vi "Mapping v10.5.0.vi"(5 "Simulate Spectra":bool, 7 "Simulate Drive":bool, 11 "Input Parameters":T6={"Drive Connection Settings"={"Objective GPIB-Port"=1, "Stage GPIB-Port"=0, "Drive Selector"=5, "Drive Velocity (V/s)"=1.0}, "ITC503 Current Values"={"ITC503 Heater"=4.0, "ITC503 Temperature"=4.0, "ITC503 P"=0.0, "ITC503 I"=5.0, "ITC503 D"=0.0, "ITC503 Setpoint"=0.0, "ITC503 Gradient"=0.0, "ITC503 Heater Auto"=FALSE, "ITC503 PID Auto"=FALSE}, "Wavelengths (nm)"=[], "Drive Current Values"={"Voltages"={"Drive X Voltage"=0.0, "Drive Y Voltage"=0.0, "Drive Z Voltage"=0.0}, "Position"={"Drive X Position"=0.0, "Drive Y Position"=0.0, "Drive Z Position"=0.0}}, "iHR Current Values"={"iHR 550 Front Entrance"=0.0, "iHR550 Side Exit"=0.0, "iHR550 Wavelength"=897.9988, "iHR550 Exit Mirror"=2, "iHR550 Grating"="1", "Grating Index"=1}, "Spectra Settings"={"Integration Time"=0.0, "Repetitions"=0, "Mapping Spectra"=TRUE}, "CCD3500 Temperature"=0.0, "Simulate Drive"=FALSE, "Simulate Spectra"=FALSE, "JYCCDLib.IJYCCDReqd"=refnum} {"Drive Connection Settings"."Drive Velocity (V/s)" min=10.0 max=160.0 step=0.1 format="%.1f"; "Drive Connection Settings"."Drive Selector" items=["Obj.", "Stage"]; "Drive Connection Settings"."Stage GPIB-Port" min=1 max=20 step=1 format="%#.0f"; "Drive Connection Settings"."Objective GPIB-Port" min=1 max=20 step=1 format="%#.0f"; "ITC503 Current Values"."ITC503 Gradient" format="%.2f"; "ITC503 Current Values"."ITC503 Setpoint" min=-273.0 max=300000.0 step=0.0001 format="%.1f"; "ITC503 Current Values"."ITC503 I" format="%_1f"; "ITC503 Current Values"."ITC503 P" format="%_1f"; "ITC503 Current Values"."ITC503 Temperature" min=0.0 max=1645.0 step=1e-05 format="%.2f"; "ITC503 Current Values"."ITC503 Heater" min=0.0 max=100.0 step=0.01 scale=0.0..100.0; "Drive Current Values"."Position"."Drive Z Position" min=-273.0 max=300000.0 step=0.0001 format="%.1f"; "Drive Current Values"."Position"."Drive Y Position" min=-273.0 max=300000.0 step=0.0001 format="%.1f"; "Drive Current Values"."Position"."Drive X Position" min=-273.0 max=300000.0 step=0.0001 format="%.1f"; "Drive Current Values"."Voltages"."Drive Z Voltage" min=-273.0 max=300000.0 step=0.0001 format="%.1f"; "Drive Current Values"."Voltages"."Drive Y Voltage" min=-273.0 max=300000.0 step=0.0001 format="%.1f"; "Drive Current Values"."Voltages"."Drive X Voltage" min=-273.0 max=300000.0 step=0.0001 format="%.1f"; "iHR Current Values"."iHR550 Exit Mirror" items=["EntranceMirror", "ExitMirror", "Front", "Side"]; "Spectra Settings"."Repetitions" min=1 max=100 step=1; "Spectra Settings"."Integration Time" min=0.5 max=6000.0 step=1.0 format="%.1f"}) -> ()   [LabVIEW 2010]
uses:
  ESA-C/TypeDefs/ESA-C Connection Settings.ctl
  TypeDefs/Mapping Spectra Params.ctl
  TypeDefs/Mapping Drive Params.ctl
  ESA-C/TypeDefs/ESA-C Set Positions.ctl
  ESA-C/TypeDefs/ESA-C Current Values.ctl
  iHR550/TypeDefs/iHR Current Values.ctl
  ITC503/TypeDefs/ITC503 Current Values.ctl
  TypeDefs/Mapping Input Parameters.ctl
  <vilib>/Utility/miscctls.llb/LVPointTypeDef.ctl
  Global Variables.vi
panel:
  out "JYCCDLib.IJYCCDReqd":refnum<k7>
  out "AutoClose":bool
  out "ITC503 Temperature":dbl caption="Sample (K)" min=10.0 max=160.0 step=0.1 format="%.1f"
  out "CCD3500 Temperature":dbl caption="CCD (°C)" min=10.0 max=160.0 step=0.1 format="%.1f"
  in  "CCD3000 Current Rep.":string="0/0"
  in  "Pause":bool
  out "Current Position":T1 {"Position"."Drive Z Position" min=-273.0 max=300000.0 step=0.0001 format="%.1f"; "Position"."Drive Y Position" min=-273.0 max=300000.0 step=0.0001 format="%.1f"; "Position"."Drive X Position" min=-273.0 max=300000.0 step=0.0001 format="%.1f"; "Voltages"."Drive Z Voltage" min=-273.0 max=300000.0 step=0.0001 format="%.1f"; "Voltages"."Drive Y Voltage" min=-273.0 max=300000.0 step=0.0001 format="%.1f"; "Voltages"."Drive X Voltage" min=-273.0 max=300000.0 step=0.0001 format="%.1f"}
  out "Target Position":T2={"Drive X Set"=10.0, "Drive Y Set"=10.0, "Drive Z Set"=10.0} {"Drive X Set" min=10.0 max=160.0 step=0.1 format="%.1f"; "Drive Z Set" min=10.0 max=160.0 step=0.1 format="%.1f"; "Drive Y Set" min=10.0 max=160.0 step=0.1 format="%.1f"}
  out "Progress":u8(slide) max=10 scale=0.0..100.0
  out "Objective Running":bool caption="Obj."
  out "CCD Running":bool caption="CCD"
  in  "Save Map":bool
  in  "Spectra Params":T3={"Integration Time"=10.0, "Repetitions"=10, "Mapping Spectra"=TRUE} {"Repetitions" min=1 max=100 step=1; "Integration Time" min=0.5 max=6000.0 step=1.0 format="%.1f"}
  in  "Drive Settings":T4={"Objective GPIB-Port"=4, "Stage GPIB-Port"=4, "Drive Selector"=0, "Drive Velocity (V/s)"=5.0} {"Drive Velocity (V/s)" min=10.0 max=160.0 step=0.1 format="%.1f"; "Drive Selector" items=["Obj.", "Stage"]; "Stage GPIB-Port" min=1 max=20 step=1 format="%#.0f"; "Objective GPIB-Port" min=1 max=20 step=1 format="%#.0f"}
  in  "Z Position":dbl caption="Z (µm)" min=0.0 max=100.0 step=0.1 format="%.1f"
  in  "Mapping Params":T5={"X Start Position"=0.0, "X Stop Position"=10.0, "Y Start Position"=0.0, "Y Stop Position"=10.0, "Step Size"=1.0} {"Step Size" min=0.1 max=30.0 step=0.1 format="%.1f"; "Y Stop Position" min=0.0 max=30.0 step=0.1 format="%.1f"; "Y Start Position" min=0.0 max=30.0 step=0.1 format="%.1f"; "X Stop Position" min=0.0 max=30.0 step=0.1 format="%.1f"; "X Start Position" min=0.0 max=30.0 step=0.1 format="%.1f"}
  in  "Exit":bool
  out "Measuring":bool
  in  "Start":bool
  out "Filename":string
  out "Full Data":dbl[][](array[numeric])
  out "Live Data":dbl[][](array[numeric])
  in  "ITC503 Current Values":T7 {"ITC503 Gradient" format="%.2f"; "ITC503 Setpoint" min=-273.0 max=300000.0 step=0.0001 format="%.1f"; "ITC503 I" format="%_1f"; "ITC503 P" format="%_1f"; "ITC503 Temperature" min=0.0 max=1645.0 step=1e-05 format="%.2f"; "ITC503 Heater" min=0.0 max=100.0 step=0.01 scale=0.0..100.0}
  in  "iHR Current Values":T8={"iHR 550 Front Entrance"=0.0, "iHR550 Side Exit"=0.0, "iHR550 Wavelength"=897.9988, "iHR550 Exit Mirror"=2, "iHR550 Grating"="1", "Grating Index"=1} {"iHR550 Exit Mirror" items=["EntranceMirror", "ExitMirror", "Front", "Side"]}
  in  "Wavelengths (nm)":dbl[](array[numeric])
  # "Status"
  # "Active"
  # "Target"
  # "Current"
  # "Parameters"
  # "Spectral"
  # "Spectral / Video Mapping"
  # "Mapping"
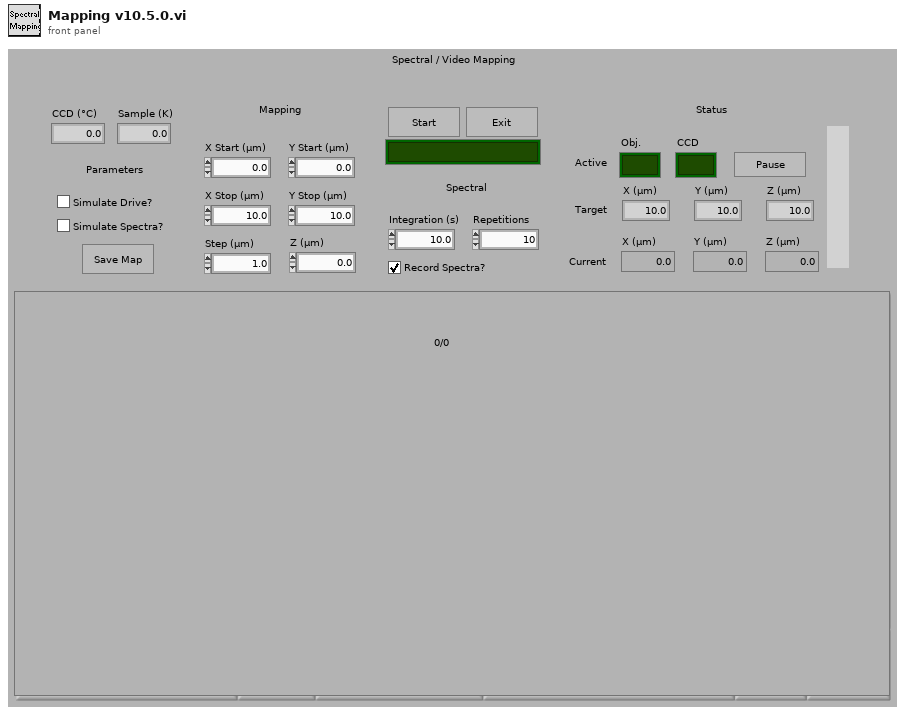
[diagram p1: front panel]
types:
  T1 = typedef "ESA-C Current Values.ctl" = cluster{"Voltages":cluster{"Drive X Voltage":dbl, "Drive Y Voltage":dbl, "Drive Z Voltage":dbl}, "Position":cluster{"Drive X Position":dbl, "Drive Y Position":dbl, "Drive Z Position":dbl}}
  T2 = typedef "ESA-C Set Positions.ctl" = cluster{"Drive X Set":dbl, "Drive Y Set":dbl, "Drive Z Set":dbl}
  T3 = typedef "Mapping Spectra Params.ctl" = cluster{"Integration Time":dbl, "Repetitions":u16, "Mapping Spectra":bool}
  T4 = typedef "ESA-C Connection Settings.ctl" = cluster{"Objective GPIB-Port":i32, "Stage GPIB-Port":i32, "Drive Selector":u16, "Drive Velocity (V/s)":dbl}
  T5 = typedef "Mapping Drive Params.ctl" = cluster{"X Start Position":dbl, "X Stop Position":dbl, "Y Start Position":dbl, "Y Stop Position":dbl, "Step Size":dbl}
  T6 = typedef "Mapping Input Parameters.ctl" = cluster{"Drive Connection Settings":T4, "ITC503 Current Values":T7, "Wavelengths (nm)":dbl[], "Drive Current Values":T1, "iHR Current Values":T8, "Spectra Settings":T3, "CCD3500 Temperature":dbl, "Simulate Drive":bool, "Simulate Spectra":bool, "JYCCDLib.IJYCCDReqd":refnum<k7>}
  T7 = typedef "ITC503 Current Values.ctl" = cluster{"ITC503 Heater":dbl, "ITC503 Temperature":dbl, "ITC503 P":dbl, "ITC503 I":dbl, "ITC503 D":dbl, "ITC503 Setpoint":dbl, "ITC503 Gradient":dbl, "ITC503 Heater Auto":bool, "ITC503 PID Auto":bool}
  T8 = typedef "iHR Current Values.ctl" = cluster{"iHR 550 Front Entrance":dbl, "iHR550 Side Exit":dbl, "iHR550 Wavelength":dbl, "iHR550 Exit Mirror":i32, "iHR550 Grating":string, "Grating Index":i32}
  T9 = typedef "LVPointTypeDef.ctl" = cluster{"Horizontal":i16, "Vertical":i16}
  T10 = typedef "NPC3SG Set Positions.ctl" = cluster{"Drive X Set":dbl, "Drive Y Set":dbl, "Drive Z Set":dbl}
  T11 = cluster{"Intensities":dbl[], "Wavelengths":dbl[]}[]
  T12 = cluster{"Intensities":dbl[], "Wavelengths":dbl[]}
  T13 = enum32{"invalid app kind", "Development System", "Run Time System", "Student Edition", "Embedded LabVIEW", "Evaluation", "Custom"}
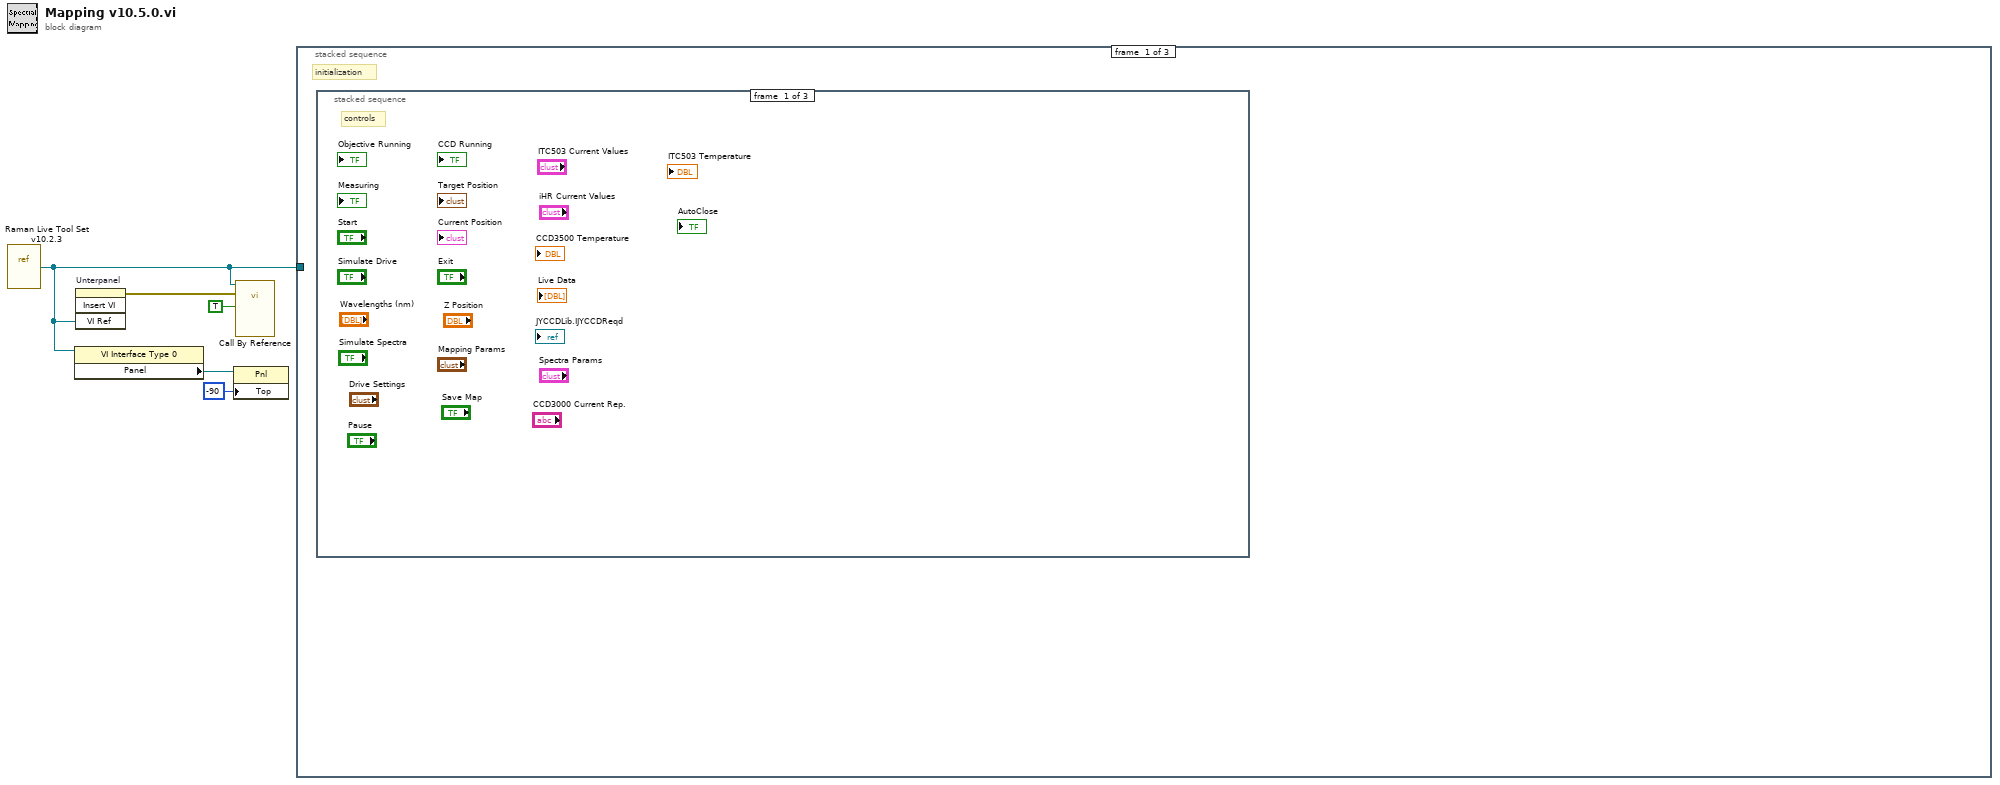
[diagram p0: block diagram]
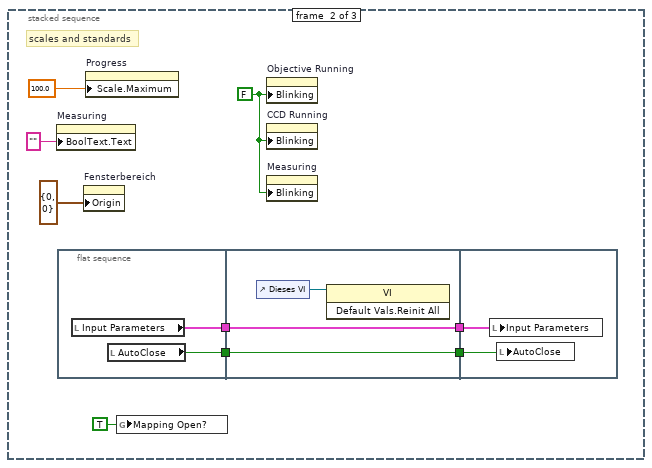
[diagram p2: hidden frame]
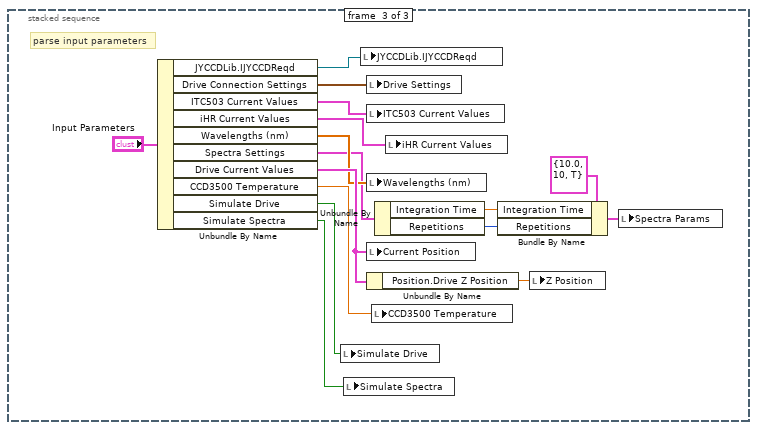
[diagram p3: hidden frame]
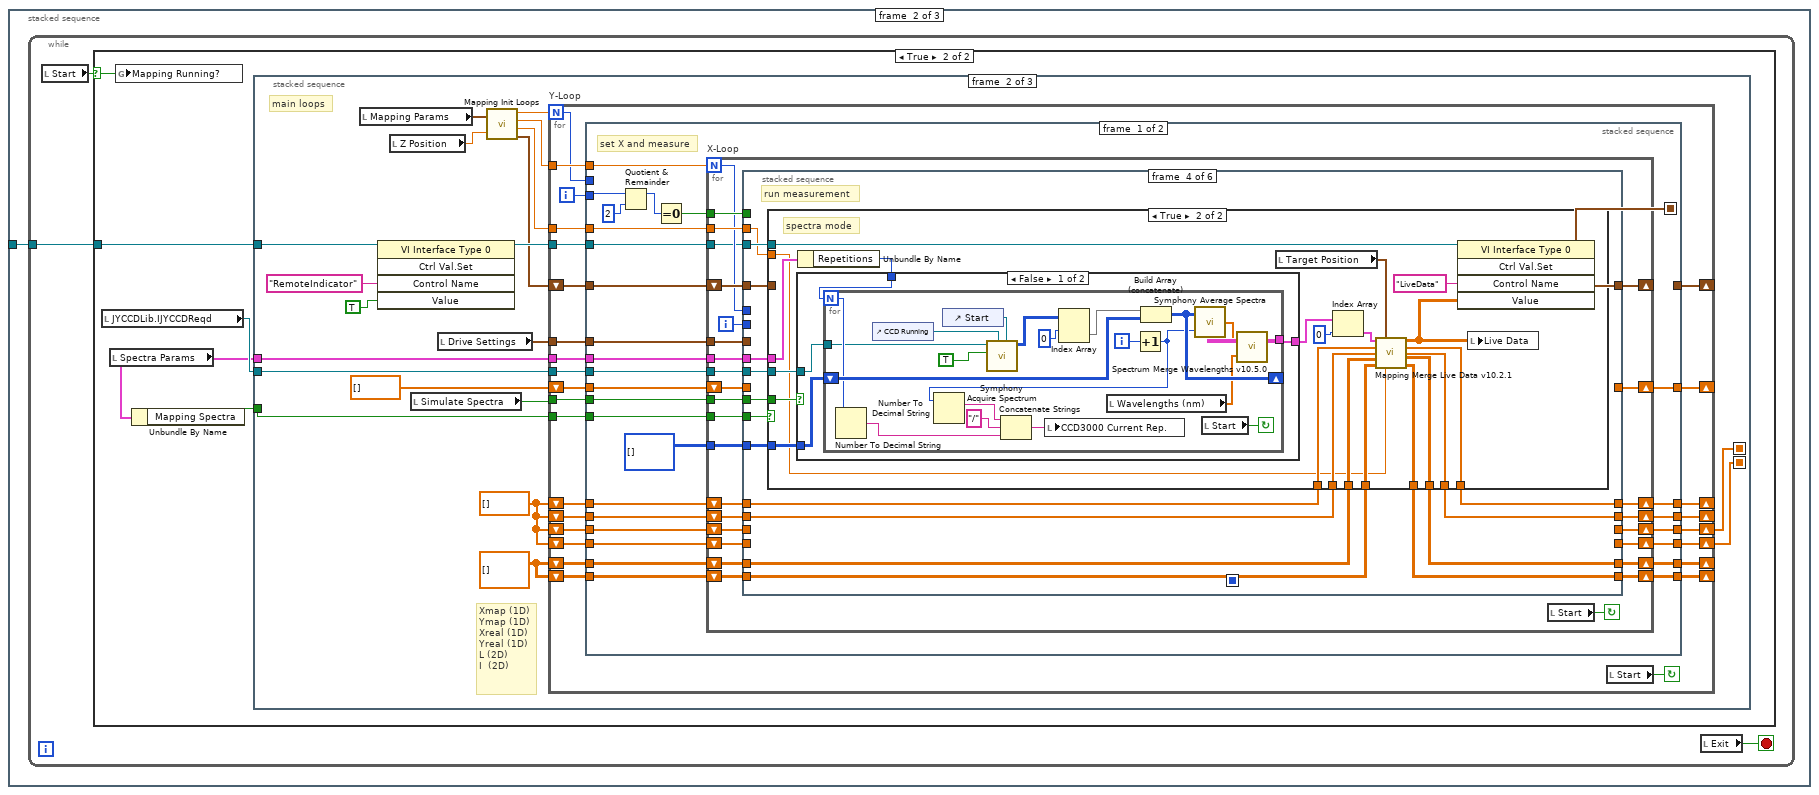
[diagram p4: hidden frame]
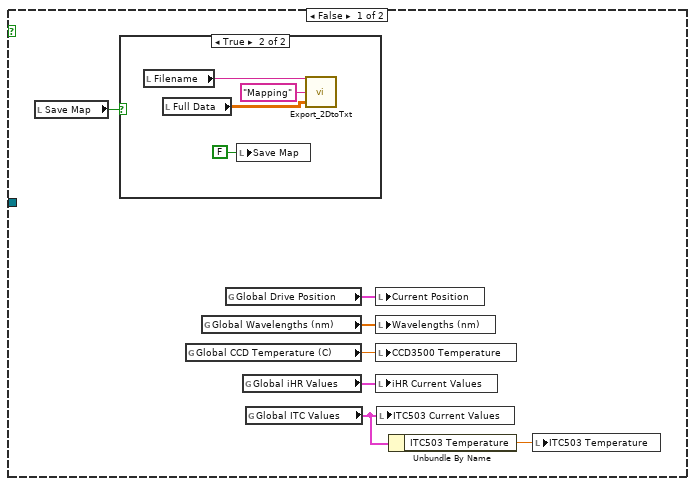
[diagram p5: hidden frame]
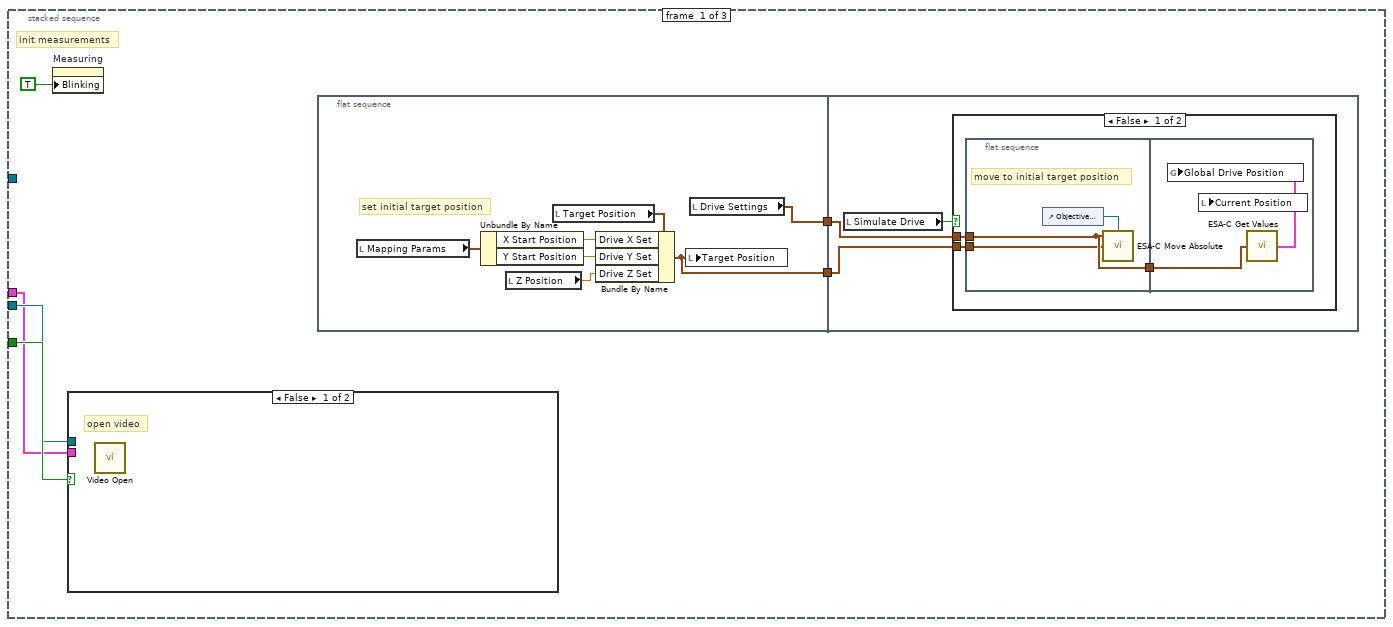
[diagram p7: hidden frame]
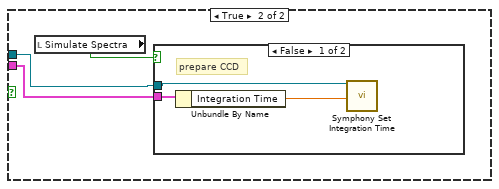
[diagram p9: hidden frame]
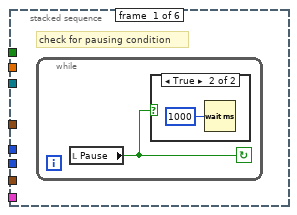
[diagram p11: hidden frame]
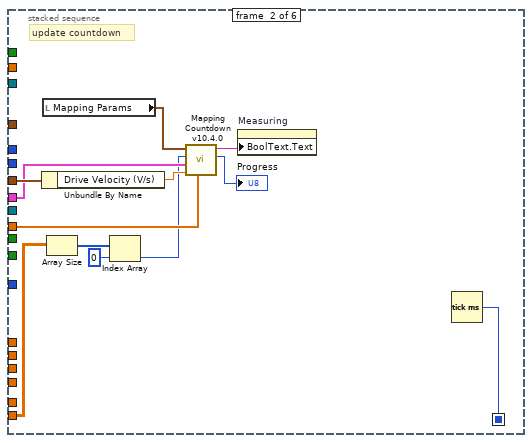
[diagram p13: hidden frame]
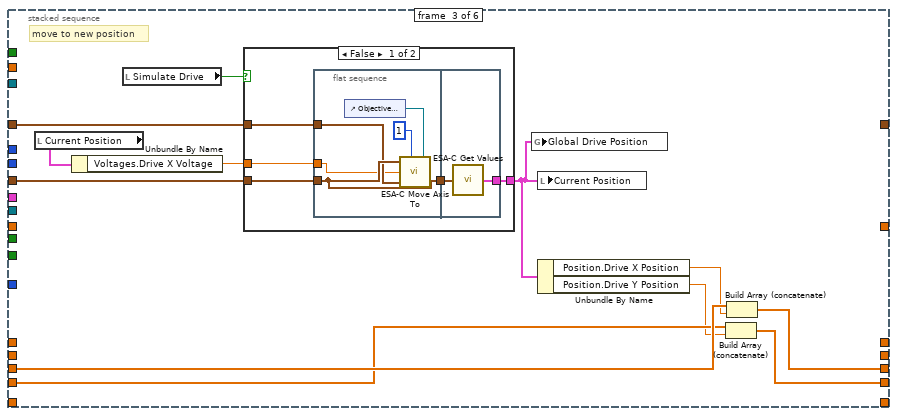
[diagram p14: hidden frame]
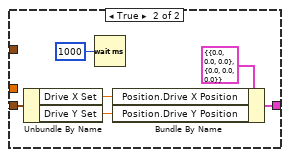
[diagram p15: hidden frame]
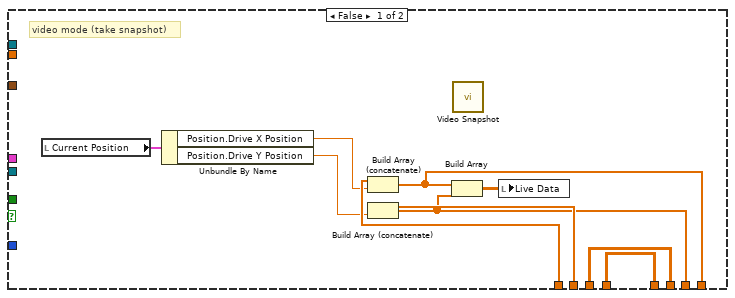
[diagram p16: hidden frame]
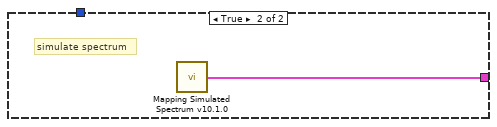
[diagram p17: hidden frame]
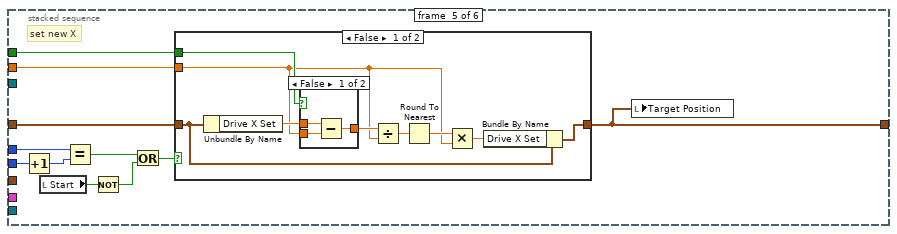
[diagram p18: hidden frame]
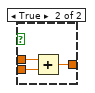
[diagram p19: hidden frame]
diagram:
  n1 = vi-ref "Raman Live Tool Set v10.2.3.vi"() -> (w3:refnum<vi>)
  n2 = property class="VI Interface Type 0"(reference=w3) -> ("Panel"=w2:refnum<vi>)  [unwired: 1 in, 2 out]
  n3 = invoke on="Unterpanel" class="Unterpanel" method="Insert VI"("VI Ref"=w3) -> (error out=w5:errorcluster)  [unwired: 3 in, 3 out]
  n4 = property class="Pnl"(reference=w2, "Top"=-90 ("Position:Oben")) -> ()  [unwired: 1 in, 2 out]
  n5 = call-by-ref "?"(reference=w3, error in=w5, "RemoteIndicator"=TRUE) -> ()  [unwired: 3 in, 2 out]
  n6 = stacked-sequence {
    tunnel: w3 -> [_ w38 w398]
    frame #0 {
      # "initialization"
      n7 = stacked-sequence {
        frame #0 {
          # "controls"
        }
        frame #1 {
          w12 = FALSE ("Blinkend")
          # "scales and standards"
          n8 = property on="Measuring" class="Bool (strict)"("BoolText.Text"="" ("Boolescher Text.Text")) -> ()  [unwired: 2 in, 2 out]
          n9 = flat-sequence {
            tunnel: [w16] -> w9
            tunnel: [w15] -> w6
            tunnel: [w18] -> w10
            tunnel: w9 -> [w18]
            tunnel: [w17] -> w7
            tunnel: w6 -> [w17]
            tunnel: w10 -> [w21]
            tunnel: w7 -> [w20]
            frame #0 {
              n10 = local read "Input Parameters"() -> (w16:T6)
              n11 = local read "AutoClose"() -> (w15:bool)
            }
            frame #1 {
              n12 = control-ref of="Dieses VI"() -> (w19:refnum<vi>)
              n13 = invoke class="VI" method="Default Vals.Reinit All"(reference=w19) -> ()  [unwired: 2 in, 3 out]
            }
            frame #2 {
              n14 = local write "Input Parameters"(w21) -> ()
              n15 = local write "AutoClose"(w20) -> ()
            }
          }
          n16 = property on="Fensterbereich" class="Pane"("Origin"=T9 {"Horizontal"=0, "Vertical"=0}) -> ()  [unwired: 2 in, 2 out]
          n17 = property on="Progress" class="Slide (strict)"("Scale.Maximum"=100.0 ("Skalierung.Bereich:Maximum")) -> ()  [unwired: 2 in, 2 out]
          n18 = global write "Global Variables.vi" "Mapping Open?"(TRUE ("Mapping Open?")) -> ()
          n19 = property on="Objective Running" class="Bool (strict)"("Blinking"=w12) -> ()  [unwired: 2 in, 2 out]
          n20 = property on="CCD Running" class="Bool (strict)"("Blinking"=w12) -> ()  [unwired: 2 in, 2 out]
          n21 = property on="Measuring" class="Bool (strict)"("Blinking"=w12) -> ()  [unwired: 2 in, 2 out]
        }
        frame #2 {
          # "parse input parameters"
          n22 = Unbundle By Name("Input Parameters") -> ("JYCCDLib.IJYCCDReqd"=w22:refnum<k7>, "Drive Connection Settings"=w35:T4, "ITC503 Current Values"=w36:T7, "iHR Current Values"=w26:T8, "Wavelengths (nm)"=w34:dbl[], "Spectra Settings"=w32:T3, "Drive Current Values"=w37:T1, "CCD3500 Temperature"=w27:dbl, "Simulate Drive"=w24:bool, "Simulate Spectra"=w23:bool)
          n23 = local write "Simulate Drive"(w24) -> ()
          n24 = local write "Simulate Spectra"(w23) -> ()
          n25 = local write "JYCCDLib.IJYCCDReqd"(w22) -> ()
          n26 = local write "Drive Settings"(w35) -> ()
          n27 = local write "ITC503 Current Values"(w36) -> ()
          n28 = local write "Wavelengths (nm)"(w34) -> ()
          n29 = local write "Current Position"(w37) -> ()
          n30 = Unbundle By Name(w37) -> ("Position.Drive Z Position"=w33:dbl)
          n31 = local write "CCD3500 Temperature"(w27) -> ()
          n32 = Unbundle By Name(w32) -> ("Integration Time"=w30:dbl, "Repetitions"=w29:u16)
          n33 = local write "iHR Current Values"(w26) -> ()
          n34 = Bundle By Name(cluster=T3 {"Integration Time"=10.0, "Repetitions"=10, "Mapping Spectra"=TRUE} ("Mapping Spectra Settings"), "Integration Time"=w30, "Repetitions"=w29) -> (w28:T3)
          n35 = local write "Z Position"(w33) -> ()
          n36 = local write "Spectra Params"(w28) -> ()
        }
      }
    }
    frame #1 {
      n37 = while {
        tunnel: w38 -> [w41]
        stop <- w40 stop-if-true
        n38 = local read "Start"() -> (w39:bool)
        n39 = case shown="True" w39 {
          selector: w39 -> [_ w53]
          tunnel: w41 -> [_ w57]
          frame False {
            n40 = local read "Save Map"() -> (w48:bool)
            n41 = case shown="True" w48 {
              frame False {
              }
              frame True {
                n42 = local read "Filename"() -> (w51:string)
                n43 = local read "Full Data"() -> (w49:dbl[][])
                n44 = local write "Save Map"(FALSE ("Save Map")) -> ()
                n45 = call "Export_2DtoTxt.vi"("Data (2D)"=w49, "Export Type"="Mapping", "Filename"=w51) -> ()  [unwired: 3 in]
              }
            }
            n46 = global read "Global Variables.vi" "Global CCD Temperature (C)"() -> (w47:dbl)
            n47 = global read "Global Variables.vi" "Global Wavelengths (nm)"() -> (w45:dbl[])
            n48 = global read "Global Variables.vi" "Global Drive Position"() -> (w46:T1)
            n49 = global read "Global Variables.vi" "Global iHR Values"() -> (w44:T8)
            n50 = global read "Global Variables.vi" "Global ITC Values"() -> (w43:T7)
            n51 = local write "Current Position"(w46) -> ()
            n52 = local write "Wavelengths (nm)"(w45) -> ()
            n53 = local write "CCD3500 Temperature"(w47) -> ()
            n54 = local write "iHR Current Values"(w44) -> ()
            n55 = local write "ITC503 Current Values"(w43) -> ()
            n56 = Unbundle By Name(w43) -> ("ITC503 Temperature"=w42:dbl)
            n57 = local write "ITC503 Temperature"(w42) -> ()
          }
          frame True {
            n58 = local read "JYCCDLib.IJYCCDReqd"() -> (w55:refnum<k7>)
            n59 = local read "Spectra Params"() -> (w54:T3)
            n60 = global write "Global Variables.vi" "Mapping Running?"(w53) -> ()
            n61 = Unbundle By Name(w54) -> ("Mapping Spectra"=w56:bool)
            n62 = stacked-sequence {
              seq-local: [_ w88 _] -> [_ _ w377]
              seq-local: [_ w89 _] -> [_ _ w376]
              tunnel: w57 -> [_ w99 _]
              tunnel: w56 -> [w62 w98 w378]
              tunnel: w54 -> [w60 w96 _]
              tunnel: w55 -> [w61 w95 _]
              frame #0 {
                # "init measurements"
                n63 = property on="Measuring" class="Bool (strict)"("Blinking"=TRUE ("Blinkend")) -> ()  [unwired: 2 in, 2 out]
                n64 = case shown="False" w62 {
                  tunnel: w61 -> [_ w84]
                  tunnel: w60 -> [_ w83]
                  frame False {
                    # "open video"
                    n65 = call "Video Open.vi"() -> ()  [unwired: 11 in, 1 out]
                  }
                  frame True {
                    n66 = local read "Simulate Spectra"() -> (w82:bool)
                    n67 = case shown="False" w82 {
                      tunnel: w84 -> [w87 _]
                      tunnel: w83 -> [w86 _]
                      frame False {
                        # "prepare CCD"
                        n68 = Unbundle By Name(w86) -> ("Integration Time"=w85:dbl)
                        n69 = call "Symphony Set Integration Time.vi"("JYCCDLib.IJYCCDReqd"=w87, "Integration (s)"=w85) -> ()  [unwired: 13 in, 1 out]
                      }
                      frame True {
                      }
                    }
                  }
                }
                n70 = flat-sequence {
                  tunnel: [w65] -> w59
                  tunnel: [w64] -> w58
                  tunnel: w59 -> [w71]
                  tunnel: w58 -> [w72]
                  frame #0 {
                    # "set initial target position"
                    n71 = local read "Mapping Params"() -> (w70:T5)
                    n72 = Unbundle By Name(w70) -> ("X Start Position"=w68:dbl, "Y Start Position"=w67:dbl)
                    n73 = local read "Z Position"() -> (w66:dbl)
                    n74 = local read "Target Position"() -> (w69:T2)
                    n75 = Bundle By Name(cluster=w69, "Drive X Set"=w68, "Drive Y Set"=w67, "Drive Z Set"=w66) -> (w65:T2)
                    n76 = local write "Target Position"(w65) -> ()
                    n77 = local read "Drive Settings"() -> (w64:T4)
                  }
                  frame #1 {
                    n78 = local read "Simulate Drive"() -> (w73:bool)
                    n79 = case shown="False" w73 {
                      tunnel: w72 -> [w76 _]
                      tunnel: w71 -> [w74 _]
                      frame False {
                        n80 = flat-sequence {
                          tunnel: w76 -> [w78]
                          tunnel: [w78] -> w75
                          tunnel: w74 -> [w77]
                          tunnel: w75 -> [w81]
                          frame #0 {
                            # "move to initial target position"
                            n81 = control-ref of="Objective Running"() -> (w79:refnum<vi>)
                            n82 = call "ESA-C Move Absolute.vi"("Running"=w79, "Drive New Abs. Positions"=w77, "Drive Connection Settings"=w78) -> ()  [unwired: 2 in]
                          }
                          frame #1 {
                            n83 = call "ESA-C Get Values.vi"("Drive Connection Settings"=w81) -> ("Drive Current Values"=w80:T1)
                            n84 = global write "Global Variables.vi" "Global Drive Position"(w80) -> ()
                            n85 = local write "Current Position"(w80) -> ()
                          }
                        }
                      }
                      frame True {
                      }
                    }
                  }
                }
              }
              frame #1 {
                w107 = dbl[][] []
                w90 = dbl[] []
                # "main loops"
                # "Xmap (1D)\nYmap (1D)\nXreal (1D)\nYreal (1D)\nL (2D)\nI  (2D)"
                n86 = local read "Mapping Params"() -> (w93:T5)
                n87 = invoke class="VI Interface Type 0" method="Ctrl Val.Set"(reference=w99, "Control Name"="RemoteIndicator" ("Elementname"), "Value"=TRUE) -> (reference out=w101:refnum<vi>)  [unwired: 2 in, 4 out]
                n88 = local read "Z Position"() -> (w92:dbl)
                n89 = local read "Simulate Spectra"() -> (w91:bool)
                n90 = local read "Drive Settings"() -> (w94:T4)
                n91 = call "Mapping Init Loops.vi"("Z Position"=w92, "Mapping Params"=w93) -> ("Start Positions"=w100:T10, "Step Size"=w102:dbl, "X Steps"=w103:dbl, "Y Steps"=w104:dbl)
                n92 = for "Y-Loop" {
                  N: w104 -> [w120]
                  tunnel: w103 -> [w133]
                  tunnel: w102 -> [w132]
                  shift-right: [w118] -> _
                  shift-left: w100 -> [w119]
                  shift-right: [w124] -> _
                  shift-left: w107 -> [w128]
                  shift-right: [w125] -> _
                  shift-left: w107 -> [w129]
                  shift-right: [w127] -> _
                  shift-left: w90 -> [w131]
                  shift-right: [w126] -> _
                  shift-left: w90 -> [w130]
                  tunnel: w101 -> [w122]
                  tunnel: w91 -> [w121]
                  tunnel: w94 -> [w117]
                  tunnel: w98 -> [w116]
                  tunnel: w96 -> [w115]
                  shift-right: [w113] -> _
                  shift-left: dbl[] [] -> [w114]
                  tunnel: w95 -> [w112]
                  shift-right: [w109] -> w89
                  shift-left: w90 -> [w110]
                  shift-right: [w108] -> w88
                  shift-left: w90 -> [w111]
                  i -> [w123]
                  stop <- w134 continue-if-true
                  n93 = stacked-sequence {
                    seq-local: [w148 _] -> [_ w349]
                    tunnel: w133 -> [w163 _]
                    tunnel: w132 -> [w162 w350]
                    tunnel: w131 -> [w161 _]
                    tunnel: w130 -> [w160 _]
                    tunnel: w129 -> [w159 _]
                    tunnel: w128 -> [w135 _]
                    tunnel: [w158 _] -> w127
                    tunnel: [w157 _] -> w126
                    tunnel: [w156 _] -> w125
                    tunnel: [w155 _] -> w124
                    tunnel: w123 -> [w152 w353]
                    tunnel: w122 -> [w150 _]
                    tunnel: w121 -> [w149 _]
                    tunnel: w120 -> [_ w351]
                    tunnel: w119 -> [w147 _]
                    tunnel: [_ w347] -> w118
                    tunnel: w117 -> [w146 w348]
                    tunnel: w116 -> [w145 _]
                    tunnel: w115 -> [w144 _]
                    tunnel: w114 -> [w143 _]
                    tunnel: [w142 _] -> w113
                    tunnel: w112 -> [w141 _]
                    tunnel: w111 -> [w139 _]
                    tunnel: w110 -> [w138 _]
                    tunnel: [w137 _] -> w109
                    tunnel: [w136 _] -> w108
                    frame #0 {
                      # "set X and measure"
                      n94 = Quotient & Remainder(x=w152, y=2) -> (x-y*floor(x/y)=w153:i32)  [unwired: 1 out]
                      n95 = Equal To 0?(x=w153) -> (x = 0?=w151:bool)
                      n96 = for "X-Loop" {
                        N: w163 -> [w177]
                        tunnel: w162 -> [w189]
                        shift-right: [w188] -> w148
                        shift-left: w147 -> [w190]
                        shift-right: [w183] -> w158
                        shift-left: w161 -> [w187]
                        shift-right: [w182] -> w157
                        shift-left: w160 -> [w186]
                        shift-right: [w180] -> w156
                        shift-left: w159 -> [w185]
                        shift-right: [w181] -> w155
                        shift-left: w135 -> [w184]
                        tunnel: w151 -> [w179]
                        tunnel: w150 -> [w176]
                        tunnel: w149 -> [w175]
                        tunnel: w146 -> [w174]
                        tunnel: w145 -> [w173]
                        tunnel: w144 -> [w172]
                        shift-right: [w171] -> w142
                        shift-left: w143 -> [w170]
                        tunnel: w141 -> [w169]
                        tunnel: u16[][] [] -> [w168]
                        shift-right: [w164] -> w136
                        shift-left: w139 -> [w167]
                        shift-right: [w165] -> w137
                        shift-left: w138 -> [w166]
                        i -> [w178]
                        stop <- w191 continue-if-true
                        n97 = stacked-sequence {
                          seq-local: [_ w198 _ _ _ _] -> [_ _ _ _ _ w338]
                          tunnel: w190 -> [_ _ w217 w251 w315 _]
                          tunnel: w189 -> [_ _ _ w236 w313 _]
                          tunnel: [_ _ _ _ w312 _] -> w188
                          tunnel: w187 -> [_ _ _ w250 _ _]
                          tunnel: w186 -> [_ _ _ w249 _ _]
                          tunnel: w185 -> [_ _ _ w247 _ _]
                          tunnel: w184 -> [_ w197 _ w248 _ _]
                          tunnel: [_ _ _ w246 _ _] -> w183
                          tunnel: [_ _ _ w245 _ _] -> w182
                          tunnel: [_ _ _ w244 _ _] -> w181
                          tunnel: [_ _ _ w243 _ _] -> w180
                          tunnel: w179 -> [_ _ _ _ w314 _]
                          tunnel: w178 -> [_ _ _ _ w318 _]
                          tunnel: w177 -> [_ _ _ _ w316 _]
                          tunnel: w176 -> [_ _ _ w242 _ _]
                          tunnel: w175 -> [_ _ _ w241 _ _]
                          tunnel: w174 -> [_ w201 w215 _ _ _]
                          tunnel: w173 -> [_ _ _ w240 _ _]
                          tunnel: w172 -> [_ w200 _ w238 _ _]
                          tunnel: [_ _ _ _ _ w335] -> w171
                          tunnel: w170 -> [_ w199 _ _ _ w337]
                          tunnel: w169 -> [_ _ _ w239 _ _]
                          tunnel: w168 -> [_ _ _ w237 _ _]
                          tunnel: w167 -> [_ _ w212 _ _ _]
                          tunnel: w166 -> [_ _ w211 _ _ _]
                          tunnel: [_ _ w208 _ _ _] -> w165
                          tunnel: [_ _ w207 _ _ _] -> w164
                          frame #0 {
                            # "check for pausing condition"
                            n98 = while {
                              stop <- w192 continue-if-true
                              n99 = local read "Pause"() -> (w192:bool)
                              n100 = case shown="True" w192 {
                                frame False {
                                }
                                frame True {
                                n101 = Wait (ms)(milliseconds to wait=u32 1000) -> ()  [unwired: 1 out]
                                }
                              }
                            }
                          }
                          frame #1 {
                            # "update countdown"
                            n102 = Unbundle By Name(w201) -> ("Drive Velocity (V/s)"=w202:dbl)
                            n103 = local read "Mapping Params"() -> (w205:T5)
                            n104 = Array Size(array=w197) -> (size(s)=w196:i32[])
                            n105 = Index Array(array=w196, index=0) -> (element=w194:i32)
                            n106 = call "Mapping Countdown v10.4.0.vi"("Execution Times (s)"=w199, "Drive Velocity"=w202, "Mapping Spectra Settings"=w200, "Ready Steps"=w194, "Mapping Drive Parameters"=w205) -> ("Progress"=→"Progress":i16, "Time String"=w203:string)  [unwired: 5 in]
                            n107 = property on="Measuring" class="Bool (strict)"("BoolText.Text"=w203) -> ()  [unwired: 2 in, 2 out]
                            n108 = Tick Count (ms)() -> (millisecond timer value=w198:u32)
                          }
                          frame #2 {
                            # "move to new position"
                            n109 = local read "Current Position"() -> (w214:T1)
                            n110 = Unbundle By Name(w214) -> ("Voltages.Drive X Voltage"=w213:dbl)
                            n111 = local read "Simulate Drive"() -> (w216:bool)
                            n112 = case shown="False" w216 {
                              tunnel: w217 -> [w221 w234]
                              tunnel: [w220 w231] -> w206
                              tunnel: w215 -> [w219 _]
                              tunnel: w213 -> [w218 _]
                              frame False {
                                n113 = flat-sequence {
                                tunnel: w221 -> [w226]
                                tunnel: [w227] -> w222
                                tunnel: w219 -> [w227]
                                tunnel: w218 -> [w223]
                                tunnel: w222 -> [w229]
                                tunnel: [w228] -> w220
                                frame #0 {
                                n114 = control-ref of="Objective Running"() -> (w224:refnum<vi>)
                                n115 = call "ESA-C Move Axis To.vi"("Drive Connection Settings"=w227, "Axis"=1, "Current Voltage (V)"=w223, "Drive New Abs. Positions"=w226, "Running"=w224) -> ()  [unwired: 2 in]
                                }
                                frame #1 {
                                n116 = call "ESA-C Get Values.vi"("Drive Connection Settings"=w229) -> ("Drive Current Values"=w228:T1)
                                }
                                }
                              }
                              frame True {
                                n117 = Unbundle By Name(w234) -> ("Drive X Set"=w235:dbl, "Drive Y Set"=w232:dbl)
                                n118 = Wait (ms)(milliseconds to wait=u32 1000 ("Zu wartende ms")) -> ()  [unwired: 1 out]
                                n119 = Bundle By Name(cluster=T1 {"Voltages"={"Drive X Voltage"=0.0, "Drive Y Voltage"=0.0, "Drive Z Voltage"=0.0}, "Position"={"Drive X Position"=0.0, "Drive Y Position"=0.0, "Drive Z Position"=0.0}} ("Drive Current Values"), "Position.Drive X Position"=w235, "Position.Drive Y Position"=w232) -> (w231:T1)
                              }
                            }
                            n120 = global write "Global Variables.vi" "Global Drive Position"(w206) -> ()
                            n121 = local write "Current Position"(w206) -> ()
                            n122 = Unbundle By Name(w206) -> ("Position.Drive X Position"=w210:dbl, "Position.Drive Y Position"=w209:dbl)
                            n123 = Build Array (concatenate)(w211, w209) -> (w208:dbl[])
                            n124 = Build Array (concatenate)(w212, w210) -> (w207:dbl[])
                          }
                          frame #3 {
                            # "run measurement"
                            n125 = case shown="True" w240 {
                              tunnel: w251 -> [_ _]
                              tunnel: w250 -> [w258 w279]
                              tunnel: w249 -> [w257 w278]
                              tunnel: w248 -> [w260 w276]
                              tunnel: w247 -> [w261 w277]
                              tunnel: [w255 w273] -> w246
                              tunnel: [w256 w272] -> w245
                              tunnel: [w260 w275] -> w244
                              tunnel: [w261 w274] -> w243
                              tunnel: w242 -> [_ w281]
                              tunnel: w241 -> [_ w280]
                              tunnel: w239 -> [_ w269]
                              tunnel: w238 -> [_ w268]
                              tunnel: w237 -> [_ w266]
                              tunnel: w236 -> [_ w262]
                              frame False {
                                # "video mode (take snapshot)"
                                n126 = local read "Current Position"() -> (w259:T1)
                                n127 = Unbundle By Name(w259) -> ("Position.Drive X Position"=w254:dbl, "Position.Drive Y Position"=w253:dbl)
                                n128 = Build Array (concatenate)(w258, w254) -> (w255:dbl[])
                                n129 = Build Array (concatenate)(w257, w253) -> (w256:dbl[])
                                n130 = Build Array(w255, w256) -> (w252:dbl[][])
                                n131 = call "Video Snapshot.vi"() -> ()  [unwired: 11 in, 1 out]
                                n132 = local write "Live Data"(w252) -> ()
                              }
                              frame True {
                                # "spectra mode"
                                n133 = Unbundle By Name(w268) -> ("Repetitions"=w267:u16)
                                n134 = case shown="False" w280 {
                                tunnel: [w285 w307] -> w265
                                tunnel: w269 -> [w286 _]
                                tunnel: w267 -> [w284 _]
                                tunnel: w266 -> [w283 _]
                                frame False {
                                n135 = for {
                                N: w284 -> [w293]
                                shift-right: [w304] -> _
                                shift-left: w283 -> [w305]
                                tunnel: [w302] -> w285
                                tunnel: w286 -> [w291]
                                i -> [w306]
                                stop <- w300 continue-if-true
                                n136 = Number To Decimal String(number=w293) -> (decimal integer string=w296:string)  [unwired: 1 in]
                                n137 = control-ref of="CCD Running"() -> (w299:refnum<vi>)
                                n138 = control-ref of="Start"() -> (w298:refnum<vi>)
                                n139 = call "Symphony Acquire Spectrum.vi"("Acquire"=w298, "Running"=w299, "ShutterOpen"=TRUE, "JYCCDLib.IJYCCDReqd"=w291) -> ("Raw Data"=w288:i32[][])  [unwired: 6 in, 1 out]
                                n140 = Index Array(array=w288, index (row)=0) -> (element=w287:i32[])  [unwired: 1 in]
                                n141 = local read "Wavelengths (nm)"() -> (w301:dbl[])
                                n142 = Increment(x=w306) -> (x+1=w292:i32)
                                n143 = Number To Decimal String(number=w292) -> (decimal integer string=w295:string)  [unwired: 1 in]
                                n144 = Concatenate Strings(w295, "/" ("string"), w296) -> (w294:string)
                                n145 = local write "CCD3000 Current Rep."(w294) -> ()
                                n146 = Build Array (concatenate)(w287, w305) -> (w304:i32[][])
                                n147 = call "Symphony Average Spectra.vi"("Repetitions"=w292, "Raw Spectra"=w304) -> ("Raw Spectrum"=w303:dbl[])
                                n148 = local read "Start"() -> (w300:bool)
                                n149 = call "Spectrum Merge Wavelengths v10.5.0.vi"("Wavelengths (nm)"=w301, "Raw Spectrum"=w303) -> ("Spectrum-Cluster"=w302:T11)  [unwired: 1 out]
                                }
                                }
                                frame True {
                                # "simulate spectrum"
                                n150 = call "Mapping Simulated Spectrum v10.1.0.vi"() -> ("Simulated Spectrum"=w307:cluster{i32[], dbl[]}[])
                                }
                                }
                                n151 = local read "Target Position"() -> (w271:T2)
                                n152 = Index Array(array=w265, index=0 ("Index")) -> (element=w264:T12)
                                n153 = call "Mapping Merge Live Data v10.2.1.vi"("New Spectrum"=w264, "Target Position"=w271, "X in (1D)"=w279, "Y in (1D)"=w278, "L in (2D)"=w277, "I in (2D)"=w276, "Step Size"=w262) -> ("Live Data"=w270:dbl[][], "X out (1D)"=w273:dbl[], "Y out (1D)"=w272:dbl[], "L out (2D)"=w274:dbl[][], "I out (2D)"=w275:dbl[][])  [unwired: 4 in]
                                n154 = invoke class="VI Interface Type 0" method="Ctrl Val.Set"(reference=w281, "Control Name"="LiveData" ("Elementname"), "Value"=w270) -> ()  [unwired: 2 in, 5 out]
                                n155 = local write "Live Data"(w270) -> ()
                              }
                            }
                          }
                          frame #4 {
                            # "set new X"
                            n156 = Increment(x=w318) -> (x+1=w317:i32)
                            n157 = local read "Start"() -> (w311:bool)
                            n158 = Equal?(x=w316, y=w317) -> (x = y?=w308:bool)
                            n159 = Not(x=w311) -> (.not. x?=w310:bool)
                            n160 = Or(x=w308, y=w310) -> (x .or. y?=w309:bool)
                            n161 = case shown="False" w309 {
                              tunnel: w315 -> [w326 w334]
                              tunnel: [w325 w334] -> w312
                              tunnel: w314 -> [w324 _]
                              tunnel: w313 -> [w319 _]
                              frame False {
                                n162 = Unbundle By Name(w326) -> ("Drive X Set"=w327:dbl)
                                n163 = case shown="False" w324 {
                                tunnel: w327 -> [w330 w332]
                                tunnel: [w329 w333] -> w320
                                tunnel: w319 -> [w328 w331]
                                frame False {
                                n164 = Subtract(x=w330, y=w328) -> (x-y=w329:dbl)
                                }
                                frame True {
                                n165 = Add(x=w332, y=w331) -> (x+y=w333:dbl)
                                }
                                }
                                n166 = Divide(x=w320, y=w319) -> (x/y=w323:dbl)
                                n167 = Round To Nearest(number=w323) -> (nearest integer value=w322:dbl)
                                n168 = Multiply(x=w322, y=w319) -> (x*y=w321:dbl)
                                n169 = Bundle By Name(cluster=w326, "Drive X Set"=w321) -> (w325:T10)
                              }
                              frame True {
                              }
                            }
                            n170 = local write "Target Position"(w312) -> ()
                          }
                          frame #5 {
                            n171 = Tick Count (ms)() -> (millisecond timer value=w339:u32)
                            n172 = Subtract(x=w339, y=w338) -> (x-y=w341:u32)
                            n173 = Divide(x=w341, y=u32 1000) -> (x/y=w336:dbl)
                            n174 = Build Array (concatenate)(w337, w336) -> (w335:dbl[])
                          }
                        }
                        n175 = local read "Start"() -> (w191:bool)
                      }
                    }
                    frame #1 {
                      # "set new Y\nand move to new position"
                      n176 = Increment(x=w353) -> (x+1=w352:i32)
                      n177 = local read "Start"() -> (w343:bool)
                      n178 = Equal?(x=w351, y=w352) -> (x = y?=w345:bool)
                      n179 = local read "Simulate Drive"() -> (w346:bool)
                      n180 = Not(x=w343) -> (.not. x?=w344:bool)
                      n181 = Or(x=w345, y=w344) -> (x .or. y?=w342:bool)
                      n182 = case shown="False" w342 {
                        tunnel: w349 -> [w374 w375]
                        tunnel: [w373 w375] -> w347
                        tunnel: w350 -> [w368 _]
                        frame False {
                          n183 = Unbundle By Name(w374) -> ("Drive Y Set"=w372:dbl)
                          n184 = Add(x=w368, y=w372) -> (x+y=w369:dbl)
                          n185 = Divide(x=w369, y=w368) -> (x/y=w370:dbl)
                          n186 = Round To Nearest(number=w370) -> (nearest integer value=w371:dbl)
                          n187 = Multiply(x=w371, y=w368) -> (x*y=w367:dbl)
                          n188 = Bundle By Name(cluster=w374, "Drive Y Set"=w367) -> (w373:T10)
                        }
                        frame True {
                        }
                      }
                      n189 = case shown="False" w346 {
                        tunnel: w348 -> [w358 _]
                        tunnel: w347 -> [w357 _]
                        frame False {
                          n190 = local read "Current Position"() -> (w356:T1)
                          n191 = Unbundle By Name(w356) -> ("Voltages.Drive Y Voltage"=w355:dbl)
                          n192 = flat-sequence {
                            tunnel: w358 -> [w360]
                            tunnel: w357 -> [w361]
                            tunnel: w355 -> [w362]
                            tunnel: [w360] -> w359
                            tunnel: [w366] -> w354
                            tunnel: w359 -> [w365]
                            frame #0 {
                              n193 = control-ref of="Objective Running"() -> (w364:refnum<vi>)
                              n194 = call "ESA-C Move Axis To.vi"("Drive Connection Settings"=w360, "Axis"=2, "Current Voltage (V)"=w362, "Drive New Abs. Positions"=w361, "Running"=w364) -> ()  [unwired: 2 in]
                            }
                            frame #1 {
                              n195 = call "ESA-C Get Values.vi"("Drive Connection Settings"=w365) -> ("Drive Current Values"=w366:T1)
                            }
                          }
                          n196 = global write "Global Variables.vi" "Global Drive Position"(w354) -> ()
                          n197 = local write "Current Position"(w354) -> ()
                        }
                        frame True {
                        }
                      }
                      n198 = local write "Target Position"(w347) -> ()
                    }
                  }
                  n199 = local read "Start"() -> (w134:bool)
                }
              }
              frame #2 {
                # "conclude measurement"
                n200 = flat-sequence {
                  tunnel: w377 -> [w385]
                  tunnel: w376 -> [w384]
                  tunnel: w378 -> [w393]
                  frame #0 {
                    # "save data"
                    n201 = global read "Global Variables.vi" "Global CCD Temperature (C)"() -> (w381:dbl)
                    n202 = global read "Global Variables.vi" "Global iHR Values"() -> (w379:T8)
                    n203 = local read "Mapping Params"() -> (w383:T5)
                    n204 = global read "Global Variables.vi" "Global ITC Values"() -> (w380:T7)
                    n205 = local read "Spectra Params"() -> (w388:T3)
                    n206 = Unbundle By Name(w383) -> ("Step Size"=w382:dbl)
                    n207 = local read "Live Data"() -> (w387:dbl[][])
                    n208 = call "Mapping Merge Real Positions v10.2.1.vi"("Live Data In"=w387, "X in (1D)"=w385, "Y in (1D)"=w384, "Step Size"=w382) -> ("Live Data Out"=w386:dbl[][])  [unwired: 11 in]
                    "Full Data" <- w386
                    n209 = call "Export_mappingFileName.vi"("ITC503 Current Values"=w380, "iHR Current Values"=w379, "Spectra Settings"=w388, "Mapping Parameters"=w383, "CCD3500 Temperature"=w381) -> ("Filename"=w389:string)
                    "Filename" <- w389
                    n210 = call "Export_2DtoTxt v10.2.0.vi"("Data (2D)"=w386, "Export Type"="Mapping", "Filename"=w389) -> ()  [unwired: 3 in]
                  }
                  frame #1 {
                    # "reset indicators"
                    n211 = case shown="False" w393 {
                      frame False {
                        n212 = call "Video Close.vi"() -> ()  [unwired: 11 in, 1 out]
                      }
                      frame True {
                      }
                    }
                    n213 = local write "Start"(FALSE ("Start")) -> ()
                    n214 = local write "CCD3000 Current Rep."("0/0" ("CCD3000 Current Rep.")) -> ()
                    n215 = global write "Global Variables.vi" "Mapping Running?"(FALSE ("Mapping Running?")) -> ()
                    n216 = property on="Measuring" class="Bool (strict)"("BoolText.Text"="" ("Boolescher Text.Text")) -> ()  [unwired: 2 in, 2 out]
                    n217 = property on="Measuring" class="Bool (strict)"("Blinking"=FALSE ("Measuring")) -> ()  [unwired: 2 in, 2 out]
                  }
                }
              }
            }
          }
        }
        n218 = local read "Exit"() -> (w40:bool)
      }
    }
    frame #2 {
      n219 = invoke class="VI Interface Type 0" method="Ctrl Val.Set"(reference=w398, "Control Name"="Exit" ("Elementname"), "Value"=TRUE) -> ()  [unwired: 2 in, 5 out]
      n220 = local read "AutoClose"() -> (w397:bool)
      n221 = flat-sequence {
        tunnel: w397 -> [w401]
        frame #0 {
          # "reset and close"
          n222 = control-ref of="Dieses VI"() -> (w404:refnum<vi>)
          n223 = global write "Global Variables.vi" "Mapping Open?"(FALSE ("Mapping Open?")) -> ()
          n224 = invoke class="VI" method="Default Vals.Reinit All"(reference=w404) -> (reference out=w402:refnum<vi>)  [unwired: 2 in, 2 out]
          n225 = property on="Measuring" class="Bool (strict)"("BoolText.Text"="" ("Boolescher Text.Text")) -> ()  [unwired: 2 in, 2 out]
          n226 = property class="App"() -> ("App.Kind"=w405:T13)  [unwired: 2 in, 2 out]
          n227 = case shown="\"Development System\"" w405 {
            tunnel: w402 -> [w407 w409]
            tunnel: w401 -> [_ w408]
            frame "invalid app kind", Default {
              n228 = invoke on="Invoke Node" class="VI" method="FP.Close"(reference=w407) -> ()  [unwired: 2 in, 3 out]
            }
            frame "Development System" {
              n229 = case shown="True" w408 {
                tunnel: w409 -> [_ w410]
                frame False {
                }
                frame True {
                  n230 = invoke on="Invoke Node" class="VI" method="FP.Close"(reference=w410) -> ()  [unwired: 2 in, 3 out]
                }
              }
            }
          }
        }
      }
    }
  }
